vi "接口状态判断.vi"(4 "IP-Port":string, 6 "客服端键":string, 8 "error in (no error)":errorcluster caption="错误输入（无错误）", 11 "MainPage 输入":refnum<class "MainPage.lvclass">) -> (0 "error out":errorcluster caption="错误输出", 1 "串口状态正常？":bool, 3 "MainPage 输出":refnum<class "MainPage.lvclass">)   [LabVIEW 2019, in "MainPage.lvlib" / "MainPage.lvclass"]
uses:
  MainPage.lvclass
panel:
  # "增加报文存储"
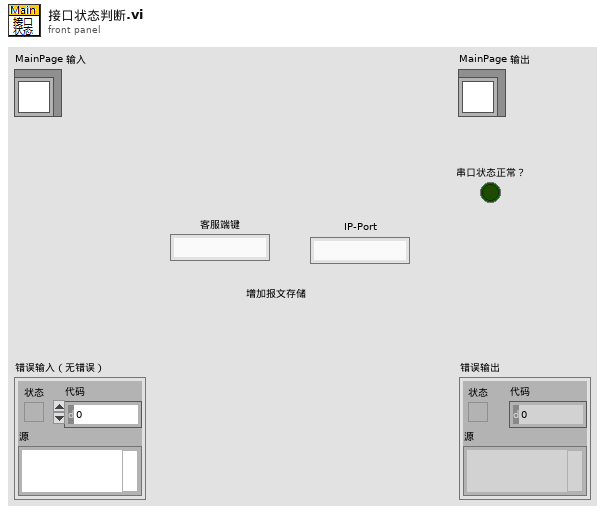
[diagram p1: front panel]
types:
  T1 = typedef "MainPage.lvlib/MainPage.lvclass/DataRef_通讯接口.ctl" = cluster{"连接方式":enum16{"网口(客服端)", "网口(服务端)", "串口"}, "VISA串口名称":refnum<visa-resource-name>, "服务端识别":cluster{"本机IP":string, "本机端口":u16, "当前目标":string, "服务端侦听ID":refnum<k5>}, "客服端识别":cluster{"客P-主IP:Port":string}, "客服端记录":map{string, refnum<k5>}, "服务端接口记录":map{string, refnum<k5>}}
  T2 = cluster{"寄存器模拟":u16[], "串口正常？":bool, "报文信息记录":string[][]}
  T3 = enum16{"ini", "增加记录", "读取记录", "更改寄存器值", "更改接口状态", "更改报文信息", "增加报文信息"}
  T4 = enum16{"ini", "读取", "写入-报文记录", "写入-寄存器模拟", "写入-串口状态", "增加报文记录"}
  T5 = cluster{"串口正常？":bool, "寄存器模拟":u16[], "报文信息记录":string[][]}
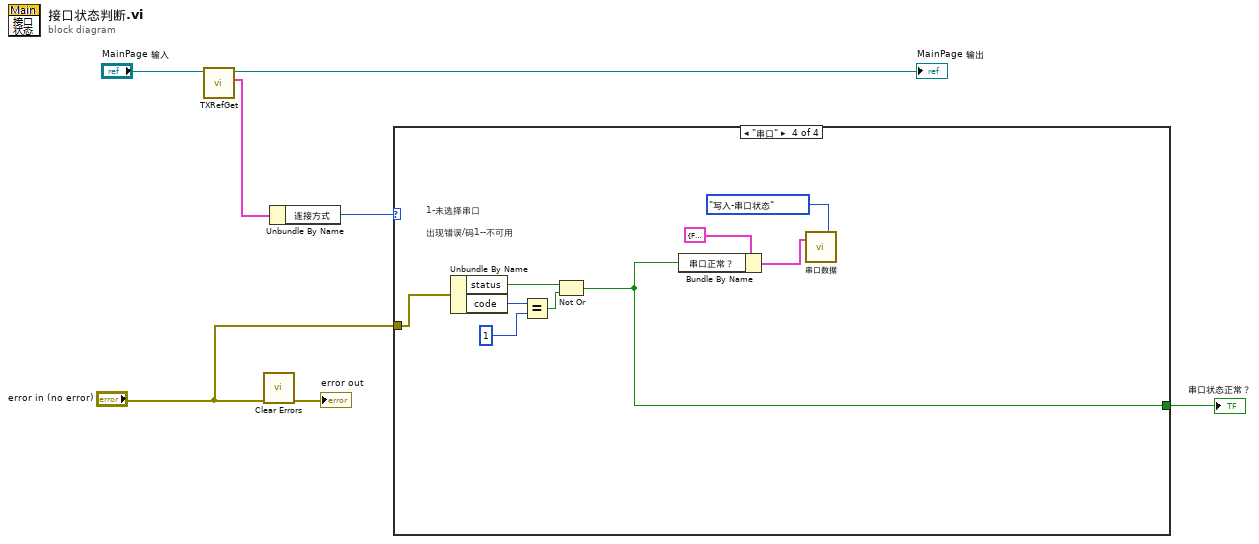
[diagram p0: block diagram]
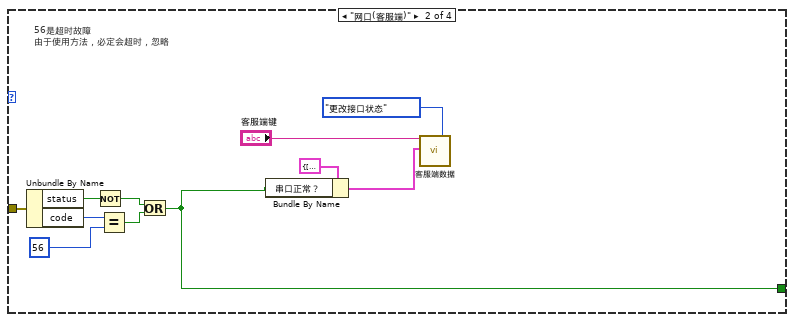
[diagram p3: hidden frame]
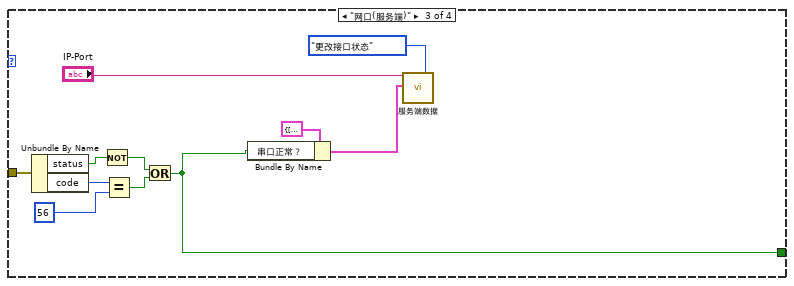
[diagram p4: hidden frame]
diagram:
  n1 = call-dynamic "TXRefGet.vi"("MainPage 输入"="MainPage 输入") -> ("通讯接口数据"=w7:T1, "MainPage 输出"=→"MainPage 输出":refnum<class "MainPage.lvclass">)  [unwired: 6 in, 3 out]
  n2 = call <vilib>:"Clear Errors.vi"("error in (no error)"="error in (no error)") -> ("error out"=→"error out":errorcluster)  [unwired: 5 in, 1 out]
  n3 = Unbundle By Name(w7) -> ("连接方式"=w6:enum16{"网口(客服端)", "网口(服务端)", "串口"})
  n4 = case shown="\"串口\"" w6 {
    tunnel: "error in (no error)" -> [_ w18 w24 w36]
    tunnel: [_ w9 w20 w31] -> w2
    frame Default {
    }
    frame "网口(客服端)" {
      # "56是超时故障\n由于使用方法，必定会超时，忽略"
      n5 = Unbundle By Name(w18) -> ("status"=w15:bool, "code"=w17:i32)
      n6 = Not(x=w15) -> (.not. x?=w14:bool)
      n7 = Equal?(x=w17, y=56) -> (x = y?=w13:bool)
      n8 = Or(x=w14, y=w13) -> (x .or. y?=w9:bool)
      n9 = Bundle By Name(cluster=T2 {"寄存器模拟"=[], "串口正常？"=FALSE, "报文信息记录"=[]} ("值"), "串口正常？"=w9) -> (w8:T2)
      n10 = call "客服端数据.vi"("客P-主IP:P"="客服端键", "数据输入"=w8, "枚举"=T3."更改接口状态") -> ()  [unwired: 15 in, 2 out]
    }
    frame "网口(服务端)" {
      n11 = Unbundle By Name(w24) -> ("status"=w27:bool, "code"=w29:i32)
      n12 = Not(x=w27) -> (.not. x?=w26:bool)
      n13 = Equal?(x=w29, y=56) -> (x = y?=w25:bool)
      n14 = Or(x=w26, y=w25) -> (x .or. y?=w20:bool)
      n15 = Bundle By Name(cluster=T2 {"寄存器模拟"=[], "串口正常？"=FALSE, "报文信息记录"=[]} ("值"), "串口正常？"=w20) -> (w21:T2)
      n16 = call "服务端数据.vi"("IP-Port"="IP-Port", "数据输入"=w21, "枚举"=T3."更改接口状态") -> ()  [unwired: 15 in, 2 out]
    }
    frame "串口" {
      # "1-未选择串口\n\n出现错误/码1--不可用"
      n17 = Unbundle By Name(w36) -> ("status"=w35:bool, "code"=w38:i32)
      n18 = Equal?(x=w38, y=1) -> (x = y?=w34:bool)
      n19 = Not Or(1:w34, 2:w35) -> (0:w31:bool)
      n20 = Bundle By Name(cluster=T5 {"串口正常？"=FALSE, "寄存器模拟"=[], "报文信息记录"=[]} ("串口反馈"), "串口正常？"=w31) -> (w30:T5)
      n21 = call "串口数据.vi"("串口输入"=w30, "枚举"=T4."写入-串口状态") -> ()  [unwired: 17 in, 1 out]
    }
  }
  "串口状态正常？" <- w2
